vi "TL_close.vi"(0 "queue DAQ":refnum<queue>, 5 "queue CAMERA":refnum<queue>, 7 "queue ASI stage":refnum<queue>, 9 "queue piezo":refnum<queue>, 11 "error in":errorcluster) -> (15 "error out":errorcluster)   [LabVIEW 2015]
uses:
  CONTROLS/Q_DAQ_element.ctl
  CONTROLS/Q_camera_element.ctl
  CONTROLS/Q_MCL_piezo_element.ctl
  CONTROLS/Q_ASI_stage_element.ctl
  GLOBAL/Global_DAQ.vi
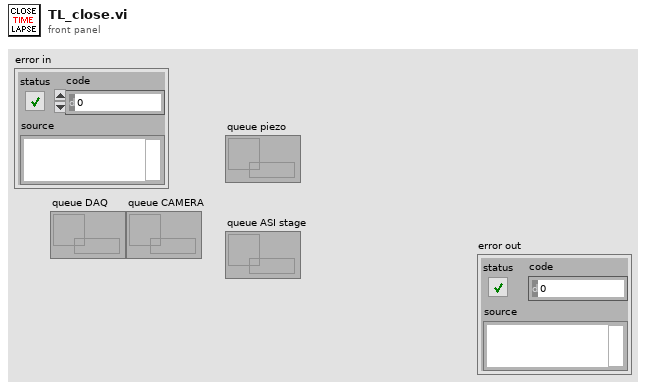
[diagram p1: front panel]
types:
  T1 = typedef "Q_DAQ_element.ctl" = cluster{"variant":variant, "Instruction":enum16{"DAQ_idle", "DAQ_initialize", "DAQ_error", "DAQ_security_stop", "DAQ_start_QPD", "DAQ_change_QPD_display", "DAQ_read_display_QPD_signal", "DAQ_QPD_init_autofocus", "DAQ_read_display_send_QPD_signal", "DAQ_close_autofocus_calibration_ramp", "DAQ_close_autofocus", "DAQ_405", "DAQ_488", "DAQ_561", "DAQ_641", "DAQ_zero_all", "DAQ_init_single_scan", "DAQ_single_scan", "DAQ_two_way_valve", "DAQ_init_merFISH", "DAQ_scan_merFISH", "DAQ_photobleaching_merFISH", "DAQ_close_merFISH", "DAQ_init_TL", "DAQ_synchro_TL", "DAQ_close_task_TL", "DAQ_close_TL", "DAQ_stop"}}
  T2 = typedef "Q_MCL_piezo_element.ctl" = cluster{"variant":variant, "Instruction":enum16{"Piezo_idle", "Piezo_initialize", "Piezo_error", "Piezo_security_stop", "Piezo_read_z", "Piezo_move_z", "Piezo_keyboard_move", "Piezo_close_autofocus_calibration_ramp", "Piezo_change_init_state", "Piezo_init_autofocus", "Piezo_init_autofocus_merFISH_TL", "Piezo_autofocus", "Piezo_autofocus_merFISH_TL", "Piezo_stop_autofocus", "Piezo_stop_autofocus_merFISH_TL", "Piezo_autofocus_lost", "Piezo_resume_autofocus_merFISH_TL", "Piezo_check_z_position_merFISH_TL", "Piezo_init_ramp", "Piezo_move_z_ramp", "Piezo_close_ramp", "Piezo_close_merFISH", "Piezo_init_TL", "Piezo_close_ramp_TL", "Piezo_close_TL", "Piezo_stop"}}
  T3 = typedef "Q_ASI_stage_element.ctl" = cluster{"variant":variant, "Instruction":enum16{"ASI_idle", "ASI_initialize", "ASI_error", "ASI_security_stop", "ASI_read_XYZ", "ASI_up", "ASI_down", "ASI_left", "ASI_right", "ASI_save_XY", "ASI_move_to_XY", "ASI_brightfield", "ASI_init_scan", "ASI_init_merFISH", "ASI_move_to_XY_merFISH", "ASI_move_to_Z_merFISH", "ASI_init_autofocus_search_merFISH", "ASI_close_autofocus_search_merFISH", "ASI_adjust_piezo_autofocus_merFISH", "ASI_set_piezo_autofocus_to_reference_position_merFISH_TL", "ASI_close_merFISH", "ASI_init_TL", "ASI_move_mosaic_TL", "ASI_brightfield_TL", "ASI_close_TL", "ASI_stop"}}
  T4 = typedef "Q_camera_element.ctl" = cluster{"variant":variant, "Instruction":enum16{"CAMERA_idle", "CAMERA_initialize", "CAMERA_error", "CAMERA_security_stop", "CAMERA_not_acquiring", "CAMERA_acquiring", "CAMERA_start_acquiring", "CAMERA_stop_acquiring", "CAMERA_change_exposure", "CAMERA_define_ROI", "CAMERA_cooler", "CAMERA_acquire_movie", "CAMERA_init_scan", "CAMERA_check_new_scan_image", "CAMERA_close_scan", "CAMERA_init_merFISH", "CAMERA_start_acquiring_merFISH", "CAMERA_close_scan_merFISH", "CAMERA_close_merFISH", "CAMERA_init_TL", "CAMERA_start_acquiring_TL", "CAMERA_stop_acquiring_TL", "CAMERA_close_TL", "CAMERA_STOP"}}
  T5 = enum16{"DAQ_idle", "DAQ_initialize", "DAQ_error", "DAQ_security_stop", "DAQ_start_QPD", "DAQ_change_QPD_display", "DAQ_read_display_QPD_signal", "DAQ_QPD_init_autofocus", "DAQ_read_display_send_QPD_signal", "DAQ_close_autofocus_calibration_ramp", "DAQ_close_autofocus", "DAQ_405", "DAQ_488", "DAQ_561", "DAQ_641", "DAQ_zero_all", "DAQ_init_single_scan", "DAQ_single_scan", "DAQ_two_way_valve", "DAQ_init_merFISH", "DAQ_scan_merFISH", "DAQ_photobleaching_merFISH", "DAQ_close_merFISH", "DAQ_init_TL", "DAQ_synchro_TL", "DAQ_close_task_TL", "DAQ_close_TL", "DAQ_stop"}
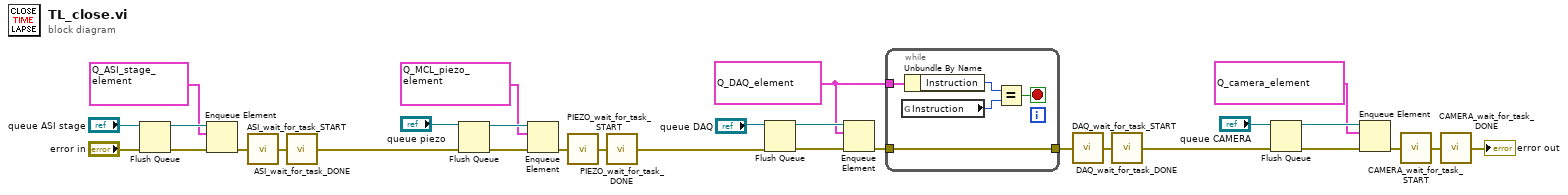
[diagram p0: block diagram]
diagram:
  w1 = T1 {"variant"=variant, "Instruction"=enum."DAQ_close_TL"} ("Q_DAQ")
  n1 = Flush Queue(queue="queue ASI stage", error in (no error)="error in") -> (queue out=w10:refnum<queue>, error out=w9:errorcluster)  [unwired: 1 out]
  n2 = Enqueue Element(queue=w10, element=T3 {"variant"=variant, "Instruction"=enum."ASI_close_TL"} ("Q_ASI_stage"), error in (no error)=w9) -> (error out=w11:errorcluster)  [unwired: 1 in, 2 out]
  n3 = call "ASI_wait_for_task_START.vi"("error in"=w11) -> ("error out"=w12:errorcluster)
  n4 = call "ASI_wait_for_task_DONE.vi"("error in"=w12) -> ("error out"=w6:errorcluster)
  n5 = Flush Queue(queue="queue piezo", error in (no error)=w6) -> (queue out=w16:refnum<queue>, error out=w18:errorcluster)  [unwired: 1 out]
  n6 = Enqueue Element(queue=w16, element=T2 {"variant"=variant, "Instruction"=enum."Piezo_close_TL"} ("Q_MCL_Piezo"), error in (no error)=w18) -> (error out=w17:errorcluster)  [unwired: 1 in, 2 out]
  n7 = call "PIEZO_wait_for_task_START.vi"("error in"=w17) -> ("error out"=w15:errorcluster)
  n8 = call "PIEZO_wait_for_task_DONE.vi"("error in"=w15) -> ("error out"=w14:errorcluster)
  n9 = Flush Queue(queue="queue DAQ", error in (no error)=w14) -> (queue out=w23:refnum<queue>, error out=w22:errorcluster)  [unwired: 1 out]
  n10 = Enqueue Element(queue=w23, element=w1, error in (no error)=w22) -> (error out=w3:errorcluster)  [unwired: 1 in, 2 out]
  n11 = while {
    tunnel: w3 -> [w32]
    tunnel: [w32] -> w2
    tunnel: w1 -> [w31]
    stop <- w34 stop-if-true
    n12 = global read "Global_DAQ.vi" "Instruction"() -> (w35:T5)
    n13 = Unbundle By Name(w31) -> ("Instruction"=w33:T5)
    n14 = Equal?(x=w33, y=w35) -> (x = y?=w34:bool)
  }
  n15 = call "DAQ_wait_for_task_START.vi"("error in"=w2) -> ("error out"=w24:errorcluster)
  n16 = call "DAQ_wait_for_task_DONE.vi"("error in"=w24) -> ("error out"=w21:errorcluster)
  n17 = Flush Queue(queue="queue CAMERA", error in (no error)=w21) -> (queue out=w28:refnum<queue>, error out=w27:errorcluster)  [unwired: 1 out]
  n18 = Enqueue Element(queue=w28, element=T4 {"variant"=variant, "Instruction"=enum."CAMERA_close_TL"} ("Q_ANDOR_element"), error in (no error)=w27) -> (error out=w29:errorcluster)  [unwired: 1 in, 2 out]
  n19 = call "CAMERA_wait_for_task_START.vi"("error in"=w29) -> ("error out"=w30:errorcluster)
  n20 = call "CAMERA_wait_for_task_DONE.vi"("error in"=w30) -> ("error out"=→"error out":errorcluster)
